vi "StopAll.vi"(1 "StepError":errorcluster, 2 "PicError":errorcluster, 3 "com in":refnum<visa-resource-name>, 4 "CmdLib In":refnum<k24>) -> (0 "错误输出":errorcluster)   [LabVIEW 2018]
uses:
  Device VIs/CmdLib.dll
  Device VIs/Verbal.vi
panel:
  out "error out":errorcluster
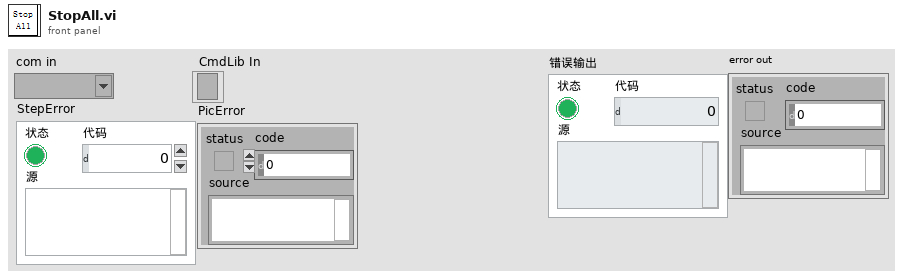
[diagram p1: front panel]
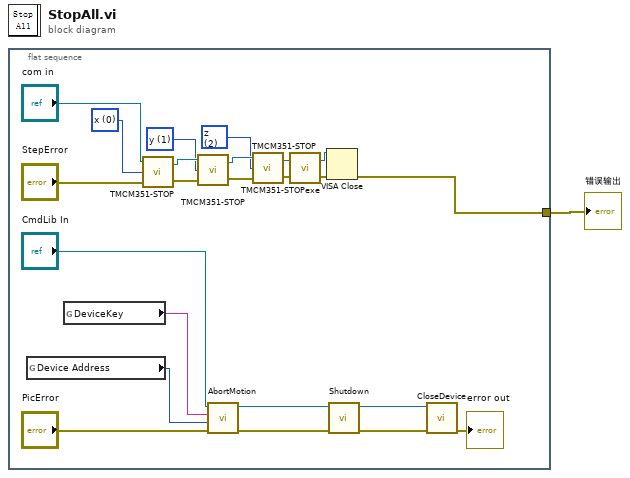
[diagram p0: block diagram]
diagram:
  n1 = flat-sequence {
    tunnel: [w3] -> w1
    frame #0 {
      w16 = u8 2 items=["x", "y", "z"] ("motor")
      w17 = u8 1 items=["x", "y", "z"] ("motor")
      w18 = u8 0 items=["x", "y", "z"] ("motor")
      n2 = global read "Verbal.vi" "Device Address"() -> (w4:i32)
      n3 = global read "Verbal.vi" "DeviceKey"() -> (w5:string)
      n4 = call "TMCM351-STOP.vi"("错误输入"="StepError", "motor"=w18, "com in"="com in") -> ("错误输出"=w21:errorcluster, "com out"=w22:refnum<visa-resource-name>)
      n5 = call "TMCM351-STOP.vi"("错误输入"=w21, "motor"=w17, "com in"=w22) -> ("错误输出"=w24:errorcluster, "com out"=w23:refnum<visa-resource-name>)
      n6 = call "AbortMotion.vi"("error in (no error)"="PicError", "Device Address In"=w4, "DeviceKey In"=w5, "CmdLib In"="CmdLib In") -> ("error out"=w12:errorcluster, "CmdLib Out"=w13:refnum<k24>)  [unwired: 2 out]
      n7 = call "TMCM351-STOP.vi"("错误输入"=w24, "motor"=w16, "com in"=w23) -> ("错误输出"=w19:errorcluster, "com out"=w20:refnum<visa-resource-name>)
      n8 = call "TMCM351-STOPexe.vi"("错误输入"=w19, "com in"=w20) -> ("错误输出"=w6:errorcluster, "com out"=w7:refnum<visa-resource-name>)
      n9 = VISA Close(VISA resource name=w7, error in (no error)=w6) -> (error out=w3:errorcluster)
      n10 = call "Shutdown.vi"("error in (no error)"=w12, "CmdLib In"=w13) -> ("error out"=w10:errorcluster, "CmdLib Out"=w11:refnum<k24>)  [unwired: 4 in]
      n11 = call "CloseDevice.vi"("error in"=w10, "CmdLib In"=w11) -> ("error out"=→"error out":errorcluster)  [unwired: 8 in, 1 out]
    }
  }
  "错误输出" <- w1
